vi "Measure.vi"(6 "error in (no error)":errorcluster, 9 "Generic Digital Multi Meter in":refnum<class "Generic Digital Multi Meter.lvclass">) -> (0 "error out":errorcluster, 2 "Array of Measurement":dbl[](array[numeric]), 3 "Generic Digital Multi Meter out":refnum<class "Generic Digital Multi Meter.lvclass">)   [LabVIEW 2016, in "Generic Digital Multi Meter.lvlib" / "Generic Digital Multi Meter.lvclass"]
uses:
  Generic Digital Multi Meter.lvclass
  Abstract Sensor/Abstract Sensor.lvclass
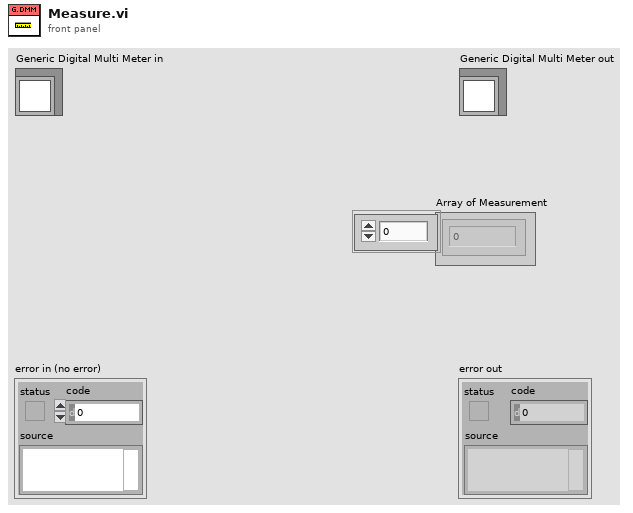
[diagram p1: front panel]
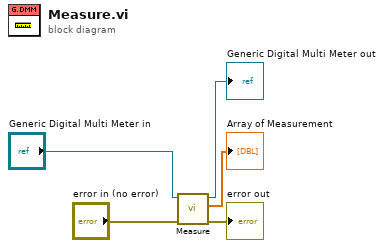
[diagram p0: block diagram]
diagram:
  n1 = call-parent "Measure.vi"("error in (no error)"="error in (no error)", "Abstract Sensor in"="Generic Digital Multi Meter in") -> ("error out"=→"error out":errorcluster, "Array of Measurement"=→"Array of Measurement":dbl[], "Abstract Sensor out"=→"Generic Digital Multi Meter out":refnum<class "Generic Digital Multi Meter.lvclass">)  [unwired: 5 in]
